vi "Receive.vi"(6 "Len":u32=8, 7 "WaitTime":i32=100, 9 "CANIndex":u32, 10 "DevIndex":u32, 11 "DevType":u32) -> (0 "VCI_CAN_OBJ":T1, 1 "CANIndex 2":u32, 2 "DevIndex 2":u32, 3 "DevType 2":u32, 4 "Len 2":u32=1, 5 "RecNUM":i32)   [LabVIEW 2016]
uses:
  ECanVci.dll
panel:
  out "添加的数组":u32[](array[numeric])
  out "WaitTime 2":i32=100
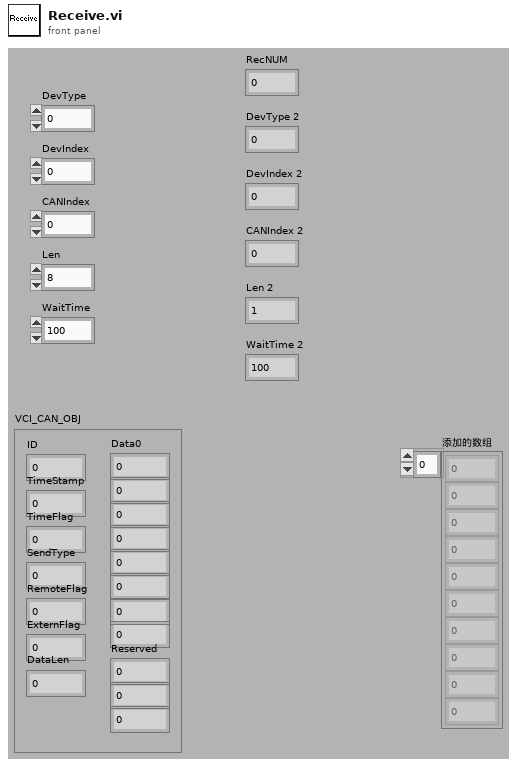
[diagram p1: front panel]
types:
  T1 = cluster{"ID":u32, "TimeStamp":u32, "TimeFlag":u8, "SendType":i8, "RemoteFlag":u8, "ExternFlag":u8, "DataLen":u8, "Data0":u8, "Data1":u8, "Data2":u8, "Data3":u8, "Data4":u8, "Data5":u8, "Data6":u8, "Data7":u8, "Reserved":u8, u8, u8}
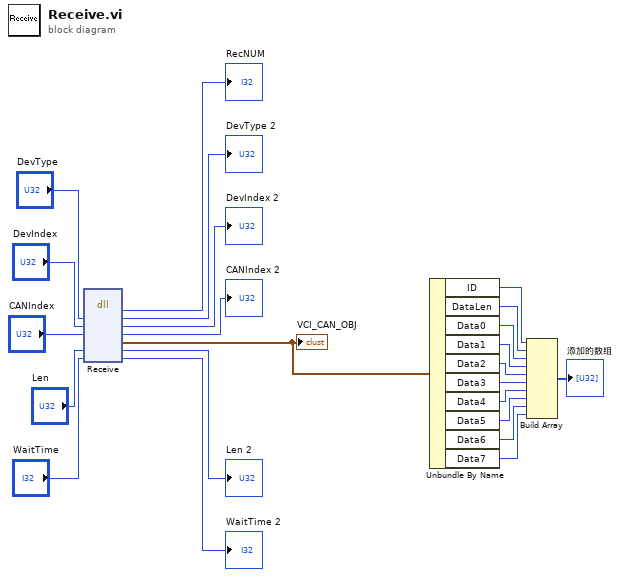
[diagram p0: block diagram]
diagram:
  n1 = dll-call lib="C:/Users/Azmat/Desktop/Labview/ECanVci.dll" fn="Receive"("DevType"="DevType", "DevIndex"="DevIndex", "CANIndex"="CANIndex", "Len"="Len", "WaitTime"="WaitTime") -> ("RecNUM"=→"RecNUM":u32, "DevType"=→"DevType 2":u32, "DevIndex"=→"DevIndex 2":u32, "CANIndex"=→"CANIndex 2":u32, "VCI_CAN_OBJ"=w12:T1, "Len"=→"Len 2":u32, "WaitTime"=→"WaitTime 2":i32)  [unwired: 3 in, 3 out]
  "VCI_CAN_OBJ" <- w12
  n2 = Unbundle By Name(w12) -> ("ID"=w11:u32, "DataLen"=w10:u8, "Data0"=w9:u8, "Data1"=w8:u8, "Data2"=w7:u8, "Data3"=w6:u8, "Data4"=w5:u8, "Data5"=w4:u8, "Data6"=w3:u8, "Data7"=w2:u8)
  n3 = Build Array(w11, w10, w9, w8, w7, w6, w5, w4, w3, w2) -> (→"添加的数组":u32[])
